vi "UHR-Fleezers Control (host) -TL FB Corrected Ronen semipassive.vi"(0 "Tab Control":T5(tab)=enum."Trap Control (RF)") -> ()   [LabVIEW 2013] (continued)
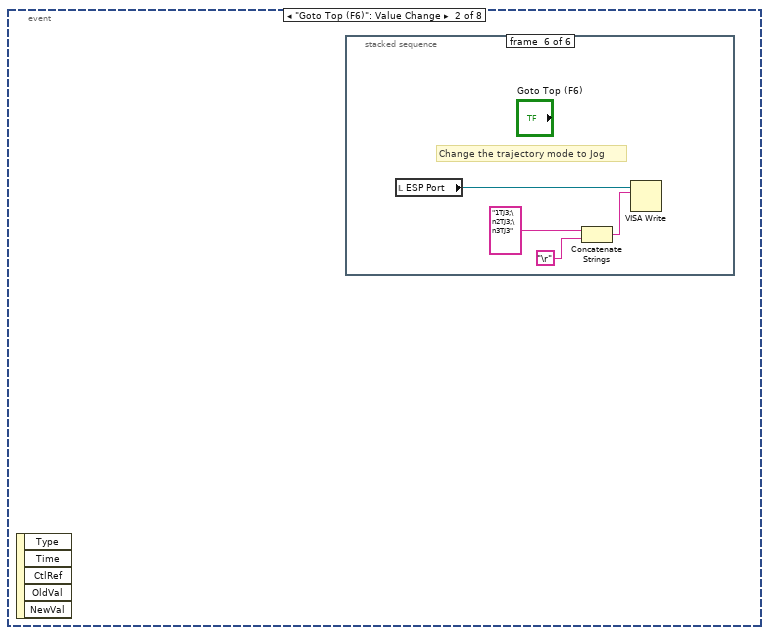
[diagram p4: hidden frame]
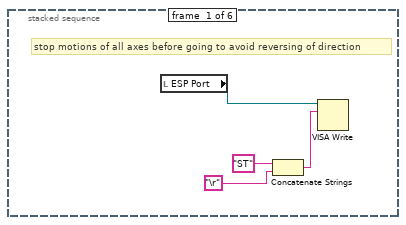
[diagram p5: hidden frame]
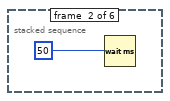
[diagram p6: hidden frame]
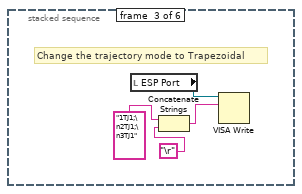
[diagram p7: hidden frame]
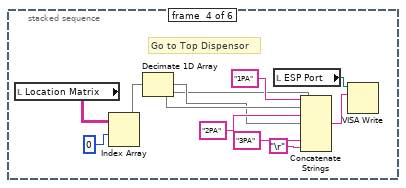
[diagram p8: hidden frame]
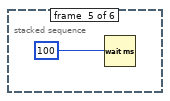
[diagram p9: hidden frame]
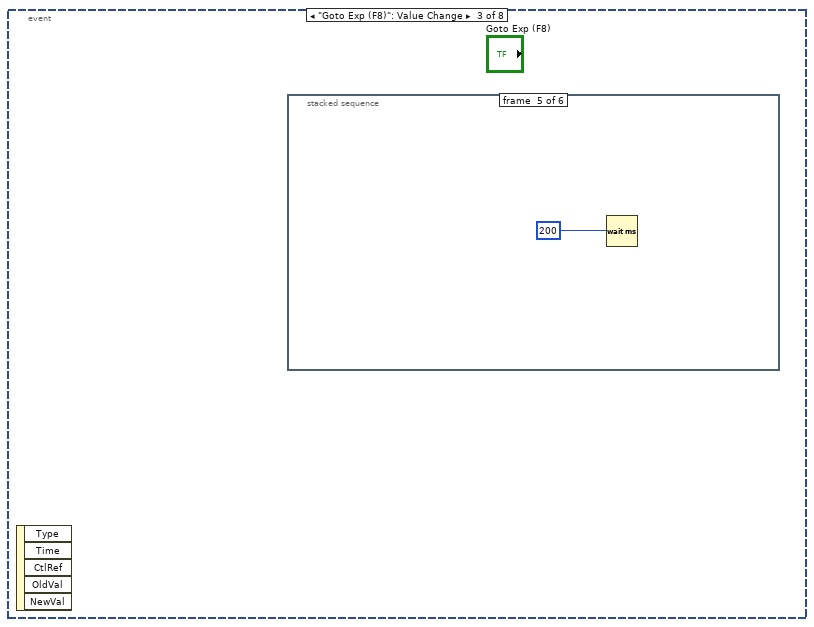
[diagram p10: hidden frame]
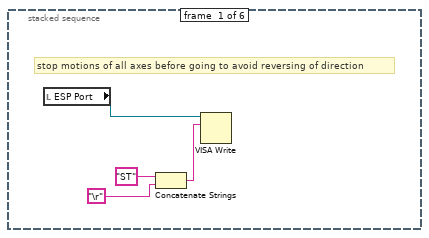
[diagram p11: hidden frame]
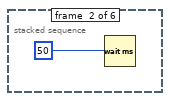
[diagram p12: hidden frame]
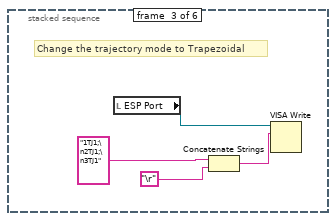
[diagram p13: hidden frame]
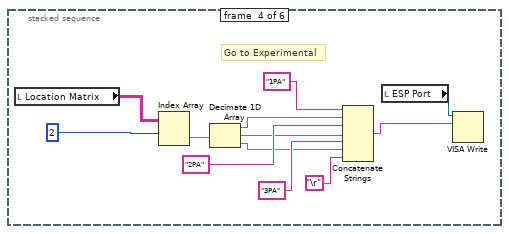
[diagram p14: hidden frame]
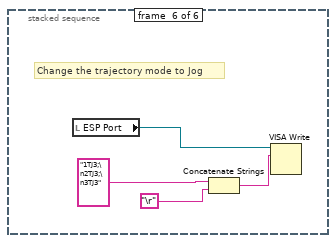
[diagram p15: hidden frame]
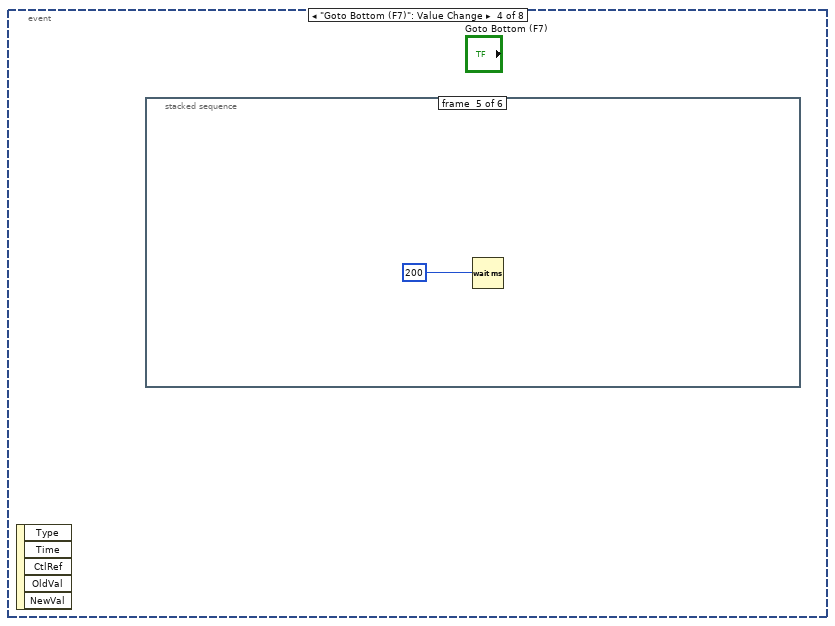
[diagram p16: hidden frame]
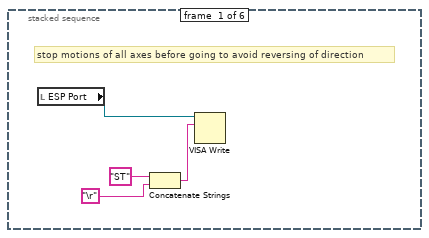
[diagram p17: hidden frame]
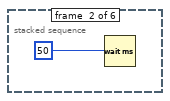
[diagram p18: hidden frame]
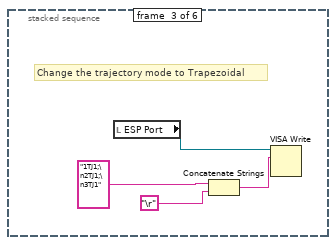
[diagram p19: hidden frame]
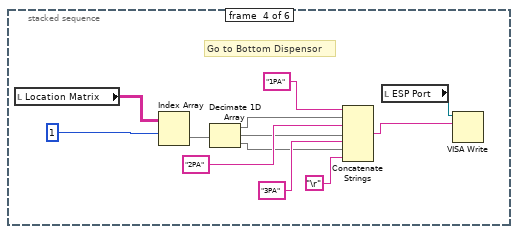
[diagram p20: hidden frame]
              frame True {
                n2315 = local write "Scan axis 2"(TRUE) -> ()
                n2316 = local write "Tether"(FALSE ("Tether")) -> ()
              }
            }
            n2317 = node-c288("Period") -> (w3831:T25)  [unwired: 3 out]
            n2318 = timed-loop "Oscillate AOD" {
              timing: w3831 -> [_]
              timing-out: [_] -> w3830
              tunnel: w3829 -> [w3841]
              tunnel: w3828 -> [w3840]
              i -> [w3843]
              stop <- w3839 stop-if-true
              n2319 = node-c288() -> (w3842:i64)  [unwired: 1 out]
              n2320 = flat-sequence {
                tunnel: w3843 -> [w3869]
                tunnel: w3842 -> [w3868]
                tunnel: w3841 -> [w3852]
                tunnel: w3840 -> [w3854]
                tunnel: [w3854] -> w3838
                tunnel: [w3853] -> w3837
                tunnel: [w3851] -> w3836
                tunnel: [w3848] -> w3834
                tunnel: w3838 -> [w3905]
                tunnel: w3837 -> [w3903]
                tunnel: w3836 -> [w3902]
                tunnel: [w3901] -> w3835
                tunnel: w3834 -> [w3900]
                tunnel: [w3969] -> w3839
                tunnel: w3835 -> [w3967]
                frame #0 {
                  n2321 = Divide(x=w3868, y=i64 1000) -> (x/y=w3863:dbl)
                  n2322 = Multiply(x=w3863, y=w3869) -> (x*y=w3865:dbl)
                  n2323 = Multiply(x="Osc. freq. (Hz)", y=6.283185307179586) -> (x*y=w3866:dbl)
                  n2324 = Multiply(x=w3866, y=w3865) -> (x*y=w3850:dbl)
                  n2325 = local read "BD 1 Frequency 2 (MHz)"() -> (w3847:dbl)
                  n2326 = local read "BD 1 Frequency 1 (MHz)"() -> (w3844:dbl)
                  n2327 = case shown="True" w3854 {
                    tunnel: w3850 -> [w3875 w3882]
                    tunnel: w3847 -> [_ w3892]
                    tunnel: [w3872 w3876] -> w3855
                    tunnel: [FALSE w3885] -> w3851
                    tunnel: [0.0 w3878] -> w3848
                    tunnel: w3844 -> [_ w3877]
                    frame False {
                      n2328 = Sine(x=w3875) -> (sin(x)=w3873:dbl)
                      n2329 = Multiply(x=w3873, y="Osc. amp. (MHz)") -> (x*y=w3872:dbl)
                    }
                    frame True {
                      n2330 = Cosine(x=w3882) -> (cos(x)=w3895:dbl)
                      n2331 = Subtract(x=w3892, y=w3877) -> (x-y=w3891:dbl)
                      n2332 = Decrement(x=w3895) -> (x-1=w3894:dbl)
                      n2333 = Subtract(x=w3891, y="Closest Delta (MHz)") -> (x-y=w3888:dbl)
                      n2334 = Divide(x=w3894, y=2.0) -> (x/y=w3889:dbl)
                      n2335 = Multiply(x=w3889, y=w3888) -> (x*y=w3876:dbl)
                      n2336 = local read "Vec Mean of T1 T2"() -> (w3884:dbl[])
                      n2337 = Greater?(x=w3884, y="Stop F (pN)") -> (0:w3886:bool[])
                      n2338 = Or Array Elements(Boolean array=w3886) -> (logical OR=w3885:bool)
                      n2339 = Divide(x=w3882, y=6.283185307179586) -> (x/y=w3881:dbl)
                      n2340 = Round Toward +Infinity(x=w3881) -> (ceil(x): smallest int >= x=w3878:dbl)
                      "Attempts" <- w3878
                      n2341 = Greater?(x=w3878, y="Attempt Limit") -> (0:w3880:bool)
                      n2342 = case shown="True" w3880 {
                        frame False {
                        }
                        frame True {
                          n2343 = local write "Fish for Tether"(FALSE ("Fish for Tether")) -> ()
                          n2344 = call <vilib>:"Beep.vi"() -> ()  [unwired: 3 in, 9 out]
                          n2345 = local read "Messages"() -> (w3897:string)
                          n2346 = call "Update messages.vi"("Message to add"="Tether fishing timeout." ("Messages"), "Old message string"=w3897) -> ("New message string"=→"Messages":string)
                        }
                      }
                    }
                  }
                  n2347 = local read "Y RF Frequency Limits (MHz)"() -> (w3856:T17)
                  n2348 = local read "X RF Frequency Limits (MHz)"() -> (w3857:T17)
                  n2349 = local read "BD 1 Frequency 3 (MHz)"() -> (w3862:dbl)
                  n2350 = local read "BD 2 Frequency 2 (MHz)"() -> (w3846:dbl)
                  n2351 = Select(t=w3847, s="Scan axis 2", f=w3846) -> (s? t:f=w3858:dbl)
                  n2352 = Add(x=w3855, y=w3858) -> (x+y=w3853:dbl)
                  n2353 = Select(t=w3853, s="Scan axis 2", f=w3847) -> (s? t:f=w3845:dbl)
                  n2354 = Select(t=w3846, s="Scan axis 2", f=w3853) -> (s? t:f=w3860:dbl)
                  n2355 = local read "BD 2 Frequency 3 (MHz)"() -> (w3861:dbl)
                  n2356 = call "set RF board frequency - interlace.vi"("Board 2 Frequency Limits"=w3856, "Board 1 Frequency Limits"=w3857, "FPGA VI Reference In"=w3852, "Board 2 Frequency 3 (MHz)"=w3861, "Board 1 Frequency 3 (MHz)"=w3862, "Board 2 Frequency 2 (MHz)"=w3846, "Board 2 Frequency 1 (MHz)"=w3860, "Board 1 Frequency 2 (MHz)"=w3845, "Board 1 Frequency 1  (MHz)"=w3844) -> ()  [unwired: 1 in, 2 out]
                }
                frame #1 {
                  n2357 = And(x=w3905, y=w3902) -> (x .and. y?=w3904:bool)
                  n2358 = case "Only if were fishing and now formed tether" shown="True" w3904 {
                    tunnel: w3903 -> [w3907 w3919]
                    tunnel: [w3906 w3918] -> w3901
                    tunnel: w3900 -> [_ w3914]
                    frame False {
                      n2359 = local read "Fish for Tether"() -> (w3906:bool)
                      n2360 = case shown="True" w3906 {
                        tunnel: w3907 -> [_ _]
                        frame False {
                        }
                        frame True {
                        }
                      }
                    }
                    frame True {
                      w3918 = FALSE ("Fish for Tether")
                      n2361 = call <vilib>:"Beep.vi"() -> ()  [unwired: 3 in, 9 out]
                      n2362 = Number To Decimal String(number=w3914, width (-)=i16 1) -> (decimal integer string=w3912:string)
                      n2363 = case shown="\"2\", \"3\", \"4\", \"5\", \"6\"" "Then..." {
                        selector: "Then..." -> [_ w3922]
                        tunnel: w3919 -> [w3921 _]
                        frame "1", Default {
                          # "do nothing"
                          n2364 = property on="BD 1 Frequency 1 (MHz)" class="DigNum (strict)"("Val(Sgnl)"=w3921) -> ()  [unwired: 2 in, 2 out]
                        }
                        frame "2", "3", "4", "5", "6" {
                          n2365 = flat-sequence {
                            tunnel: w3922 -> [w3924]
                            frame #0 {
                              n2366 = property on="Trap Delta (MHz)" class="DigNum (strict)"("Val(Sgnl)"="Move to Delta 1 (MHz)") -> ()  [unwired: 2 in, 2 out]
                            }
                            frame #1 {
                              n2367 = case shown="\"5\", \"6\"" w3924 {
                                selector: w3924 -> [w3927 w3937 _]
                                frame "3", "4" {
                                n2368 = flat-sequence {
                                tunnel: w3927 -> [w3928]
                                tunnel: [w3928] -> w3925
                                tunnel: [w3930] -> w3926
                                tunnel: w3925 -> [w3930]
                                tunnel: w3926 -> [w3934]
                                frame #0 {
                                n2369 = property on="Green Laser ON/Interlacing" class="Bool (strict)"("Val(Sgnl)"=TRUE ("Value (Signaling)")) -> ()  [unwired: 2 in, 2 out]
                                }
                                frame #1 {
                                n2370 = Multiply(x="Wait Before Save (s)", y=u32 1000 ("x")) -> (x*y=w3932:u32)
                                n2371 = Wait (ms)(milliseconds to wait=w3932) -> ()  [unwired: 1 out]
                                }
                                frame #2 {
                                n2372 = property on="Start Saving" class="Bool (strict)"("Value"=TRUE ("Start Saving")) -> ()  [unwired: 2 in, 2 out]
                                n2373 = case shown="Default" w3934 {
                                frame Default {
                                }
                                frame "4" {
                                n2374 = property on="Fl. Triggered..." class="Bool (strict)"("Val(Sgnl)"=TRUE ("Value (Signaling)")) -> ()  [unwired: 2 in, 2 out]
                                }
                                }
                                }
                                }
                                }
                                frame "5", "6" {
                                n2375 = stacked-sequence {
                                tunnel: w3937 -> [_ _ _ _ _ _ _ _ w3954 _ _]
                                frame #0 {
                                n2376 = Replace Array Subset(array=u32[] [0] ("Index Values"), new element="Raster Set Upon Tether", index=0) -> (w3938:u32[])
                                n2377 = property on="Saved AOD Raster Scan Parameter Sets" class="Arr (strict)"("Index Values"=w3938) -> ()  [unwired: 2 in, 2 out]
                                }
                                frame #1 {
                                n2378 = Wait (ms)(milliseconds to wait=u32 500) -> ()  [unwired: 1 out]
                                }
                                frame #2 {
                                n2379 = property on="Load parameters" class="Bool (strict)"("Val(Sgnl)"=TRUE ("Value (Signaling)")) -> ()  [unwired: 2 in, 2 out]
                                }
                                frame #3 {
                                n2380 = Wait (ms)(milliseconds to wait=u32 500) -> ()  [unwired: 1 out]
                                }
                                frame #4 {
                                n2381 = property on="Trap Raster Scan" class="Bool (strict)"("Val(Sgnl)"=TRUE ("Value (Signaling)")) -> ()  [unwired: 2 in, 2 out]
                                }
                                frame #5 {
                                n2382 = Wait (ms)(milliseconds to wait=u32 2000) -> ()  [unwired: 1 out]
                                }
                                frame #6 {
                                n2383 = while {
                                stop <- w3949 stop-if-true
                                n2384 = local read "Raster Scanning..."() -> (w3948:bool)
                                n2385 = local read "Saving..."() -> (w3951:bool)
                                n2386 = Wait (ms)(milliseconds to wait=u32 100) -> ()  [unwired: 1 out]
                                n2387 = Not(x=w3951) -> (.not. x?=w3950:bool)
                                n2388 = Not(x=w3948) -> (.not. x?=w3947:bool)
                                n2389 = And(x=w3950, y=w3947) -> (x .and. y?=w3949:bool)
                                }
                                }
                                frame #7 {
                                n2390 = property on="Trap Delta (MHz)" class="DigNum (strict)"("Val(Sgnl)"="Move to Delta 2 (MHz)") -> ()  [unwired: 2 in, 2 out]
                                }
                                frame #8 {
                                n2391 = local read "Tether"() -> (w3955:bool)
                                n2392 = case shown="True" w3955 {
                                tunnel: w3954 -> [_ w3956]
                                frame False {
                                }
                                frame True {
                                n2393 = flat-sequence {
                                tunnel: w3956 -> [w3958]
                                frame #0 {
                                n2394 = Wait (ms)(milliseconds to wait=u32 500) -> ()  [unwired: 1 out]
                                }
                                frame #1 {
                                n2395 = case shown="\"6\"" w3958 {
                                frame Default {
                                }
                                frame "6" {
                                n2396 = property on="Green Laser ON/Interlacing" class="Bool (strict)"("Val(Sgnl)"=TRUE ("Green Laser ON/Interlacing")) -> ()  [unwired: 2 in, 2 out]
                                }
                                }
                                }
                                frame #2 {
                                n2397 = Wait (ms)(milliseconds to wait=u32 500) -> ()  [unwired: 1 out]
                                }
                                frame #3 {
                                n2398 = local write "Start Saving"("Save at end (5, 6)") -> ()
                                }
                                }
                                }
                                }
                                }
                                frame #9 {
                                n2399 = local read "Bead Sep. Int. Time (s)"() -> (w3964:dbl)
                                n2400 = Multiply(x=w3964, y=1000.0) -> (x*y=w3963:dbl)
                                n2401 = Wait (ms)(milliseconds to wait=w3963) -> ()  [unwired: 1 out]
                                }
                                frame #10 {
                                n2402 = property on="Rescale on Mean" class="Bool (strict)"("Val(Sgnl)"=TRUE ("Value (Signaling)")) -> ()  [unwired: 2 in, 2 out]
                                }
                                }
                                }
                                frame "2", Default {
                                }
                              }
                            }
                          }
                        }
                      }
                      n2403 = Concatenate Strings("Formed tether in ", w3912, " attempt(s)." ("string")) -> (w3909:string)
                      n2404 = local read "Messages"() -> (w3916:string)
                      n2405 = local write "Fish for Tether"(w3918) -> ()
                      n2406 = call "Update messages.vi"("Message to add"=w3909, "Old message string"=w3916) -> ("New message string"=w3915:string)
                      n2407 = local write "Messages"(w3915) -> ()
                      n2408 = Get Date/Time In Seconds() -> (seconds since 1Jan1904=→"Time tether formed":timestamp)
                      "Tether" <- "Tether Alarm?"
                    }
                  }
                }
                frame #2 {
                  n2409 = local read "Oscillate Set 2"() -> (w3968:bool)
                  n2410 = local read "Stop All"() -> (w3970:bool)
                  n2411 = Not Or(1:w3967, 2:w3968) -> (0:w3966:bool)
                  n2412 = Compound Arithmetic op=OR(w3970, w3966) -> (w3969:bool)
                }
              }
              n2413 = node-c288() -> ()  [unwired: 2 out]
            }
            n2414 = node-c288(w3830) -> ()  [unwired: 1 out]
          }
        }
      }
      event "Fl. Triggered...": Value Change {
        n2415 = event-data() -> ()  [unwired: 7 out]
        n2416 = case shown="True" "Fl. Triggered..." {
          frame False {
          }
          frame True {
            n2417 = node-c288() -> (w3982:T25)  [unwired: 4 out]
            n2418 = timed-loop {
              timing: w3982 -> [_]
              timing-out: [_] -> w3981
              tunnel: "Action" -> [w3986]
              shift-right: [w3983] -> _
              shift-left: u8 255 -> [w3985]
              stop <- w3987 stop-if-true
              n2419 = node-c288() -> ()  [unwired: 2 out]
              n2420 = flat-sequence {
                tunnel: w3986 -> [w3999]
                tunnel: w3985 -> [w3996]
                tunnel: [w3995] -> w3984
                tunnel: [w4085] -> w3987
                tunnel: w3984 -> [w4084]
                tunnel: [w4084] -> w3983
                frame #0 {
                  n2421 = local read "Delta Fl. 2"() -> (w3990:dbl)
                  n2422 = local read "Delta Fl. 1"() -> (w3991:dbl)
                  n2423 = Select(t=w3991, s="APD to Watch", f=w3990) -> (s? t:f=w3989:dbl)
                  n2424 = Multiply(x="Fl. Delta Thresh. (kHz)", y=1000.0) -> (x*y=w3998:dbl)
                  n2425 = Greater?(x=w3989, y=w3998) -> (0:w3993:bool)
                  n2426 = Or(x="Force Yank", y=w3993) -> (x .or. y?=w3994:bool)
                  n2427 = case shown="True" w3994 {
                    tunnel: w3999 -> [_ w4009]
                    tunnel: w3996 -> [w4001 w4005]
                    tunnel: [w4001 w4002] -> w3995
                    frame False {
                    }
                    frame True {
                      n2428 = flat-sequence {
                        tunnel: w4006 -> [w4015]
                        tunnel: [w4015] -> w4010
                        tunnel: w4009 -> [w4014]
                        tunnel: [w4014] -> w4008
                        tunnel: [w4013] -> w4007
                        tunnel: w4005 -> [w4012]
                        tunnel: [w4011] -> w4004
                        tunnel: w4010 -> [w4040]
                        tunnel: w4008 -> [w4039]
                        tunnel: w4007 -> [w4038]
                        tunnel: w4004 -> [w4037]
                        tunnel: [w4037] -> w4003
                        tunnel: w4003 -> [w4082]
                        tunnel: [w4082] -> w4002
                        frame #0 {
                          n2429 = call <vilib>:"Beep.vi"() -> ()  [unwired: 3 in, 9 out]
                          n2430 = local write "Waiting"(FALSE ("Waiting")) -> ()
                          n2431 = Increment(x=w4012) -> (x+1=w4011:u8)
                          n2432 = case shown="\"Yank\"" w4014 {
                            tunnel: w4011 -> [_ _ w4021]
                            frame "Image" {
                              n2433 = property on="Confocal Image" class="Bool (strict)"("Val(Sgnl)"=TRUE ("Value (Signaling)")) -> ()  [unwired: 2 in, 2 out]
                            }
                            frame "Alarm", Default {
                            }
                            frame "Yank" {
                              n2434 = flat-sequence {
                                tunnel: w4021 -> [w4024]
                                tunnel: [w4023] -> w4020
                                tunnel: ["N Array El"] -> w4019
                                tunnel: w4020 -> [w4034]
                                tunnel: w4019 -> [w4030]
                                frame #0 {
                                n2435 = Multiply(x="Yank Delay (s)", y=1000.0) -> (x*y=w4027:dbl)
                                n2436 = Quotient & Remainder(x=w4024, y="N Array El") -> (x-y*floor(x/y)=w4023:u8)  [unwired: 1 out]
                                n2437 = Wait (ms)(milliseconds to wait=w4027) -> ()  [unwired: 1 out]
                                }
                                frame #1 {
                                n2438 = Random Number (0-1)() -> (number: 0 to 1=w4031:dbl)
                                n2439 = Multiply(x=w4030, y=w4031) -> (x*y=w4029:dbl)
                                n2440 = Round Toward -Infinity(1:w4029) -> (0:w4028:dbl)
                                n2441 = Select(t=w4028, s="Random Choice", f=w4034) -> (s? t:f=w4032:dbl)
                                n2442 = Index Array(array="Yank to Delta Array (MHz)", index=w4032) -> (element=w4035:dbl)
                                n2443 = property on="Trap Delta (MHz)" class="DigNum (strict)"("Val(Sgnl)"=w4035) -> ()  [unwired: 2 in, 2 out]
                                }
                              }
                            }
                          }
                          n2444 = local read "Time (s)"() -> (w4013:dbl)
                          "Fl. High" <- TRUE ("Yanking")
                        }
                        frame #1 {
                          n2445 = node-c288() -> (w4042:T25)  [unwired: 4 out]
                          n2446 = timed-loop {
                            timing: w4042 -> [_]
                            timing-out: [_] -> w4041
                            tunnel: w4040 -> [w4058]
                            tunnel: w4039 -> [w4056]
                            tunnel: w4038 -> [w4055]
                            stop <- w4057 stop-if-true
                            n2447 = node-c288() -> ()  [unwired: 2 out]
                            n2448 = local read "Fl. Delta Thresh. (kHz)"() -> (w4050:dbl)
                            n2449 = local read "Fl. Triggered..."() -> (w4059:bool)
                            n2450 = local read "Delta Fl. 1"() -> (w4046:dbl)
                            n2451 = local read "Delta Fl. 2"() -> (w4044:dbl)
                            n2452 = local read "Stop All"() -> (w4053:bool)
                            n2453 = local read "APD to Watch"() -> (w4045:bool)
                            n2454 = Select(t=w4046, s=w4045, f=w4044) -> (s? t:f=w4043:dbl)
                            n2455 = Not(x=w4059) -> (.not. x?=w4054:bool)
                            n2456 = Multiply(x=w4050, y=1000.0) -> (x*y=w4049:dbl)
                            n2457 = Negate(x=w4049) -> (-x=w4048:dbl)
                            n2458 = Less?(x=w4043, y=w4048) -> (x < y?=w4052:bool)
                            n2459 = Compound Arithmetic op=OR(w4052, w4053, w4054, "Force Reset") -> (w4057:bool)
                            n2460 = case shown="True" w4057 {
                              tunnel: w4058 -> [_ w4070]
                              tunnel: w4056 -> [_ w4069]
                              tunnel: w4055 -> [_ w4067]
                              frame False {
                              }
                              frame True {
                                n2461 = case shown="\"Yank\"" w4069 {
                                tunnel: w4070 -> [_ w4071]
                                frame "Image", Default {
                                }
                                frame "Yank" {
                                n2462 = flat-sequence {
                                tunnel: [w4076] -> w4072
                                tunnel: w4071 -> [w4076]
                                tunnel: w4072 -> [w4077]
                                frame #0 {
                                n2463 = local read "Yank Delay (s)"() -> (w4075:dbl)
                                n2464 = Multiply(x=w4075, y=1000.0) -> (x*y=w4073:dbl)
                                n2465 = Wait (ms)(milliseconds to wait=w4073) -> ()  [unwired: 1 out]
                                }
                                frame #1 {
                                n2466 = property on="Trap Delta (MHz)" class="DigNum (strict)"("Val(Sgnl)"=w4077) -> ()  [unwired: 2 in, 2 out]
                                }
                                }
                                }
                                }
                                n2467 = local read "Time (s)"() -> (w4068:dbl)
                                n2468 = Subtract(x=w4068, y=w4067) -> (x-y=w4064:dbl)
                                "Duration (s)" <- w4064
                                n2469 = Number To Decimal String(number=w4064, width (-)=i16 0) -> (decimal integer string=w4062:string)
                                n2470 = Concatenate Strings(w4062, " s fluorescence event." ("string")) -> (w4060:string)
                                n2471 = local read "Messages"() -> (w4066:string)
                                n2472 = call "Update messages.vi"("Message to add"=w4060, "Old message string"=w4066) -> ("New message string"=w4065:string)
                                n2473 = call <vilib>:"Beep.vi"() -> ()  [unwired: 3 in, 9 out]
                                n2474 = local write "Messages"(w4065) -> ()
                              }
                            }
                            n2475 = node-c288() -> ()  [unwired: 2 out]
                          }
                          n2476 = node-c288(w4041) -> ()  [unwired: 1 out]
                        }
                        frame #2 {
                          n2477 = local write "Fl. High"(FALSE ("Yanking")) -> ()
                        }
                      }
                      n2478 = local read "Trap Delta (MHz)"() -> (w4006:dbl)
                    }
                  }
                }
                frame #1 {
                  n2479 = local read "Stop All"() -> (w4088:bool)
                  n2480 = local read "Fl. Triggered..."() -> (w4086:bool)
                  n2481 = Not(x=w4086) -> (.not. x?=w4087:bool)
                  n2482 = Or(x=w4087, y=w4088) -> (x .or. y?=w4085:bool)
                  n2483 = Not(x=w4085) -> (.not. x?=→"Waiting":bool)
                }
              }
              n2484 = node-c288() -> ()  [unwired: 2 out]
            }
            n2485 = node-c288(w3981) -> ()  [unwired: 1 out]
          }
        }
      }
      event "Stop All": Value Change {
        n2486 = event-data() -> ()  [unwired: 7 out]
        n2487 = local read "Stop All"() -> (w4094:bool)
      }
    }
    n2488 = node-c288() -> ()  [unwired: 2 out]
  }
  n2489 = node-c288(w93) -> ()  [unwired: 1 out]
  n2490 = node-c288(w181) -> ()  [unwired: 1 out]
  n2491 = flat-sequence {
    tunnel: w53 -> [w4099]
    tunnel: [w4098] -> w59
    tunnel: [w4095] -> w58
    tunnel: w57 -> [_]
    tunnel: w56 -> [_]
    tunnel: w55 -> [_]
    tunnel: w54 -> [_]
    tunnel: w52 -> [w4096]
    tunnel: w59 -> [w4102]
    tunnel: w58 -> [w4101]
    frame #0 {
      w4097 = FALSE ("APD to FIFO")
      n2492 = xnode "Read/Write Control"("FPGA VI Reference In"=w4099, "error in"=w4096, "APD to FIFO"=w4097, "AI to FIFO"=w4097) -> ("FPGA VI Reference Out"=w4098:T20, "error out"=w4095:errorcluster)
    }
    frame #1 {
      n2493 = xnode "Invoke Method"("FPGA VI Reference In"=w4102, "error in"=w4101) -> ("FPGA VI Reference Out"=w4100:T20)  [unwired: 1 out]
      n2494 = xnode "Close FPGA VI Reference"("FPGA VI Reference In"=w4100) -> ()  [unwired: 1 in, 1 out]
    }
  }
